vi "Lineup Log.vi"   [LabVIEW 2014]
uses:
  Begin/Global RefNums.vi
  <vilib>/Rock Robotics/WPI/Ultrasonic/WPI_SonarMB1010AnalogRefNum Registry Get.vi
  Begin/Global Variables.vi
  <vilib>/Rock Robotics/WPI/Ultrasonic/WPI_SonarMB1010AnalogGetRange.vi
types:
  T1 = typedef "WPI_SonarMB1010AnalogDeviceRef.ctl" = cluster{"AIDeviceRef":T2, "Scaling factor (V/in)":dbl, "Average Bits":u8}
  T2 = typedef "WPI_AnalogChannelDevRef.ctl" = cluster{"DevStatus":errorcluster, "Controller":T3, "Analog Channel":T4}
  T3 = typedef "FPGA_TypedefAnalogModule.ctl" = enum16{"Controller 1"}
  T4 = typedef "FPGA_AIChannel.ctl" = enum8{"AI 0", "AI 1", "AI 2", "AI 3", "AI MXP 0", "AI MXP 1", "AI MXP 2", "AI MXP 3", "Invalid"}
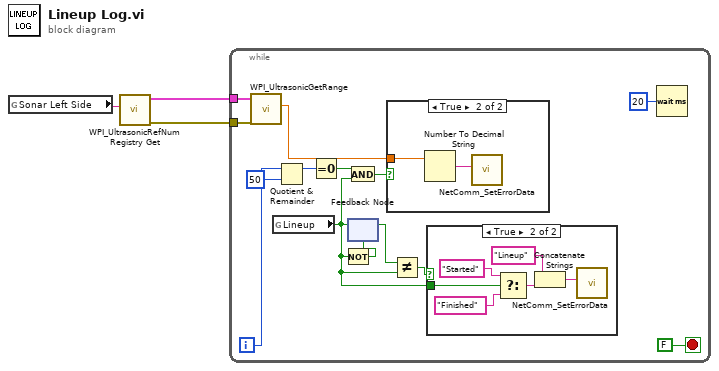
[diagram p0: block diagram]
diagram:
  n1 = global read "Global RefNums.vi" "Sonar Left Side"() -> (w3:string)
  n2 = call-poly <vilib>:"WPI_UltrasonicRefNum Registry Get.vi"("refnum name"=w3) -> ("error out"=w1:errorcluster, "SonarMB1010AnalogDevRef"=w2:T1)  [unwired: 9 in]
  n3 = while {
    tunnel: w2 -> [w17]
    tunnel: w1 -> [w16]
    i -> [w5]
    stop <- FALSE ("stop") stop-if-true
    n4 = call-poly <vilib>:"WPI_UltrasonicGetRange.vi"("error in"=w16, "SonarMB1010AnalogDevRef"=w17) -> ("Distance"=w15:dbl)  [unwired: 7 in, 2 out]
    n5 = global read "Global Variables.vi" "Lineup"() -> (w8:bool)
    n6 = Quotient & Remainder(x=w5, y=50) -> (x-y*floor(x/y)=w6:i32)  [unwired: 1 out]
    n7 = Equal To 0?(x=w6) -> (x = 0?=w7:bool)
    n8 = Not(x=w8) -> (.not. x?=w13:bool)
    n9 = And(x=w7, y=w8) -> (x .and. y?=w9:bool)
    n10 = feedback #1(w13) -> (w14:bool)
    n11 = feedback-in #1(w8) -> ()
    n12 = case shown="True" w9 {
      tunnel: w15 -> [_ w24]
      frame False {
      }
      frame True {
        n13 = Number To Decimal String(number=w24) -> (decimal integer string=w25:string)  [unwired: 1 in]
        n14 = call <vilib>:"NetComm_SetErrorData.vi"("Error Data"=w25) -> ()  [unwired: 3 in, 8 out]
      }
    }
    n15 = Not Equal?(x=w14, y=w8) -> (x != y?=w12:bool)
    n16 = case shown="True" w12 {
      tunnel: w8 -> [_ w23]
      frame False {
      }
      frame True {
        n17 = Select(t="Started" ("string"), s=w23, f="Finished" ("string")) -> (s? t:f=w20:string)
        n18 = Concatenate Strings("Lineup" ("string"), w20) -> (w19:string)
        n19 = call <vilib>:"NetComm_SetErrorData.vi"("Error Data"=w19) -> ()  [unwired: 3 in, 8 out]
      }
    }
    n20 = Wait (ms)(milliseconds to wait=u32 20) -> ()  [unwired: 1 out]
  }
